vi "GetTrendPointProps.vi"(7 "data event":T1, 9 "hw status":string, 10 "found hw status":bool, 11 "DataSetName":string) -> (3 "key value pairs out":T7[](array[typedef]))   [LabVIEW 2017, in "McsaDataEventCreator.lvlib"]
uses:
  <vilib>/addons/InsightCM/Devices/Shared/Mcsa/McsaDataEventCreator/McsaDataEventCreator.lvlib
  <vilib>/addons/InsightCM/MessageBus/Base/controls/KeyValuePair.ctl
  <vilib>/addons/InsightCM/Devices/Shared/Mcsa/McsaDataEventCreator/controls/DataEventConfig.ctl
  <vilib>/addons/InsightCM/Devices/Shared/Mcsa/McsaDataEventCreator/controls/AcqParams.ctl
  <vilib>/addons/InsightCM/Devices/Shared/Common/DataAccumulator/controls/AccumulationSettings.ctl
  <vilib>/addons/InsightCM/Devices/Shared/Common/DataAccumulator/controls/accumulationType.ctl
  <vilib>/addons/InsightCM/Devices/Shared/Common/DVRBuffer/controls/BufferLocation.ctl
  <vilib>/addons/PointValueMap/controls/PointMap.ctl
  <vilib>/addons/InsightCM/Utilities/PropertyHelpers/PropertyHelpers.lvlib
  <vilib>/addons/InsightCM/Devices/Shared/Common/DataEventCreator/DataEventCreator.lvlib
  <vilib>/addons/InsightCM/Devices/Shared/Common/DataAccumulator/DataAccumulator.lvlib
  <vilib>/addons/InsightCM/Devices/Shared/Common/DVRBuffer/DVRBuffer.lvlib
  <vilib>/addons/PointValueMap/PointValueMap.lvlib
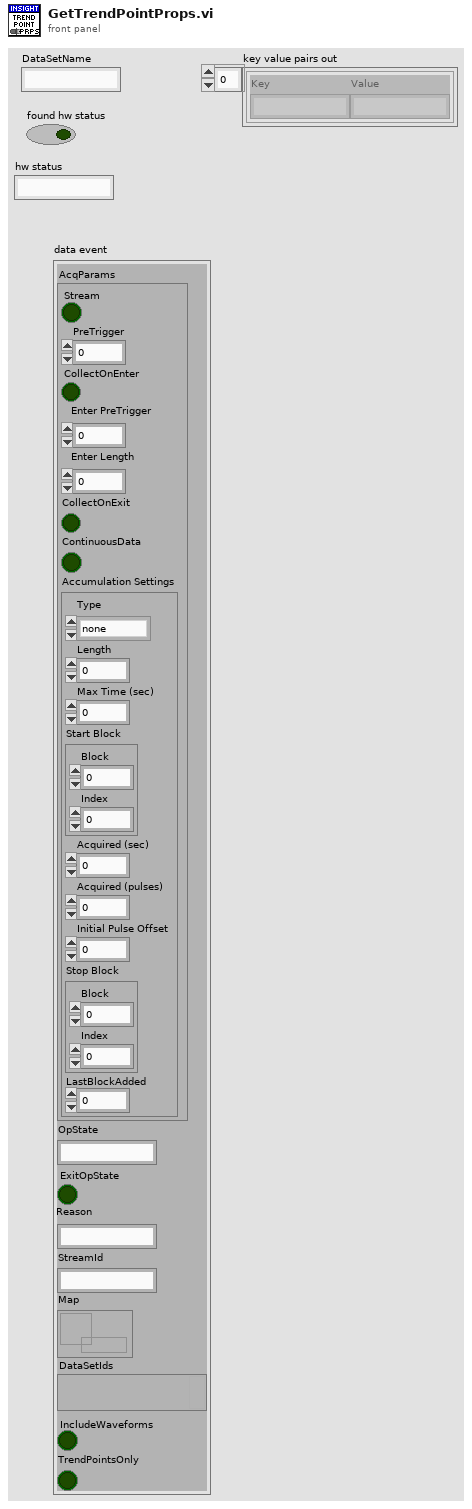
[diagram p1: front panel]
types:
  T1 = typedef "McsaDataEventCreator.lvlib/DataEventConfig.ctl" = cluster{"AcqParams":T2, "OpState":string, "ExitOpState":bool, "Reason":string, "StreamId":string, "Map":T6, "DataSetIds":variant, "IncludeWaveforms":bool, "TrendPointsOnly":bool}
  T2 = typedef "McsaDataEventCreator.lvlib/AcqParams.ctl" = cluster{"Stream":bool, "PreTrigger":i32, "CollectOnEnter":bool, "Enter PreTrigger":i32, "Enter Length":dbl, "CollectOnExit":bool, "ContinuousData":bool, "Accumulation Settings":T3}
  T3 = typedef "DataAccumulator.lvlib/AccumulationSettings.ctl" = cluster{"Type":T4, "Length":dbl, "Max Time (sec)":dbl, "Start Block":T5, "Acquired (sec)":dbl, "Acquired (pulses)":i32, "Initial Pulse Offset":dbl, "Stop Block":T5, "LastBlockAdded":u32}
  T4 = typedef "DataAccumulator.lvlib/accumulationType.ctl" = enum16{"none", "seconds", "revolutions"}
  T5 = typedef "DVRBuffer.lvlib/BufferLocation.ctl" = cluster{"Block":u32, "Index":i32}
  T6 = typedef "PointValueMap.lvlib/PointMap.ctl" = refnum<data-value>
  T7 = typedef "KeyValuePair.ctl" = cluster{"Key":string, "Value":string}
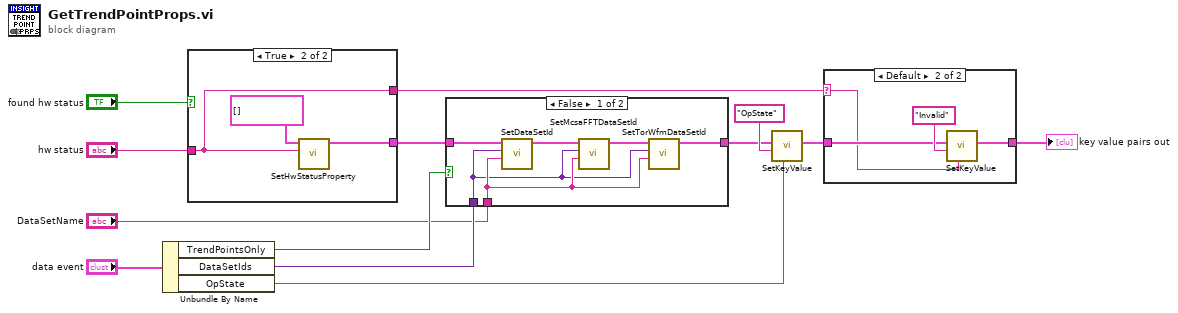
[diagram p0: block diagram]
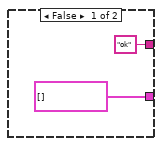
[diagram p4: hidden frame]
diagram:
  n1 = Unbundle By Name("data event") -> ("TrendPointsOnly"=w6:bool, "DataSetIds"=w4:variant, "OpState"=w8:string)
  n2 = case shown="True" "found hw status" {
    tunnel: [T7[] [] ("props out") w18] -> w12
    tunnel: "hw status" -> [_ w16]
    tunnel: ["ok" ("hw status") w16] -> w1
    frame False {
    }
    frame True {
      n3 = call <vilib>:"SetHwStatusProperty.vi"("hw status"=w16, "props in"=T7[] []) -> ("props out"=w18:T7[])  [unwired: 9 in]
    }
  }
  n4 = case shown="False" w6 {
    tunnel: w12 -> [w24 w25]
    tunnel: [w21 w25] -> w10
    tunnel: "DataSetName" -> [w20 _]
    tunnel: w4 -> [w19 _]
    frame False {
      n5 = call <vilib>:"SetDataSetId.vi"("DataSetName"=w20, "DataSetIds"=w19, "props in"=w24) -> ("props out"=w23:T7[])  [unwired: 8 in]
      n6 = call <vilib>:"SetMcsaFFTDataSetId.vi"("DataSetName"=w20, "DataSetIds"=w19, "props in"=w23) -> ("props out"=w22:T7[])  [unwired: 8 in]
      n7 = call <vilib>:"SetTorWfmDataSetId.vi"("DataSetName"=w20, "DataSetIds"=w19, "props in"=w22) -> ("props out"=w21:T7[])  [unwired: 8 in]
    }
    frame True {
    }
  }
  n8 = call <vilib>:"SetKeyValue.vi"("value"=w8, "key"="OpState", "key value pairs"=w10) -> ("key value pairs out"=w2:T7[])  [unwired: 8 in]
  n9 = case shown="Default" w1 {
    selector: w1 -> [_ w27]
    tunnel: [w26 w30] -> w5
    tunnel: w2 -> [w26 w28]
    frame "ok" {
    }
    frame Default {
      n10 = call <vilib>:"SetKeyValue.vi"("value"=w27, "key"="Invalid", "key value pairs"=w28) -> ("key value pairs out"=w30:T7[])  [unwired: 8 in]
    }
  }
  "key value pairs out" <- w5
